vi "Set_reference_Point (SubVI).vi"(7 "Part of multigrid":bool, 8 "error in (no error)":errorcluster, 11 "Application in":refnum<vi>) -> (0 "error out":errorcluster, 3 "Application out":refnum<vi>)   [LabVIEW 2021]
uses:
  <userlib>/Nanonis Prog Interface V5/Nanonis Prog Interface.lvlib
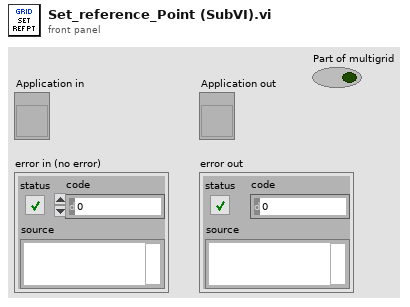
[diagram p1: front panel]
types:
  T1 = cluster{"x(m)":sgl, "y(m)":sgl, "Text":string, "Color":u32}
  T2 = cluster{"X (m)":sgl, "Y (m)":sgl, "Text":string, "Color":u32, "Visible":bool}[]
  T3 = cluster{"X (m)":sgl, "Y (m)":sgl, "Text":string, "Color":u32, "Visible":bool}
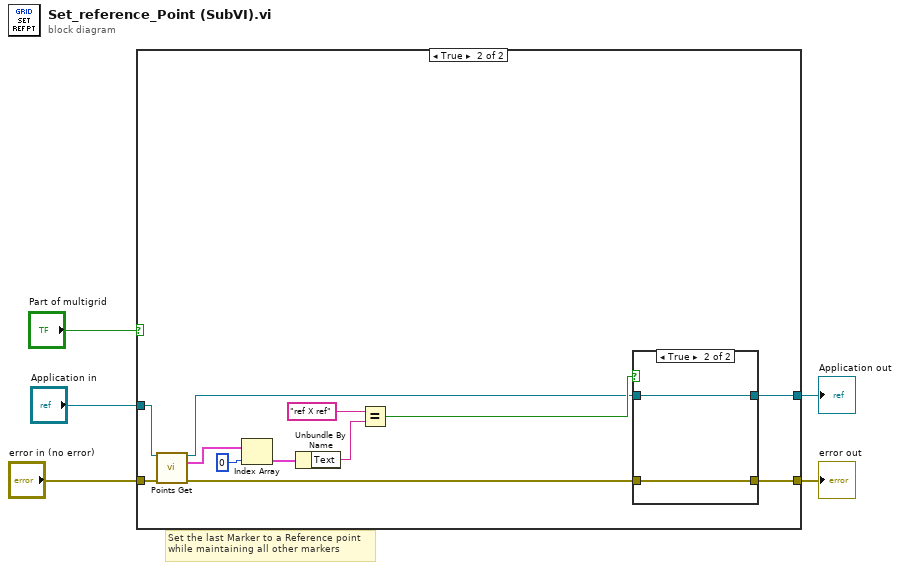
[diagram p0: block diagram]
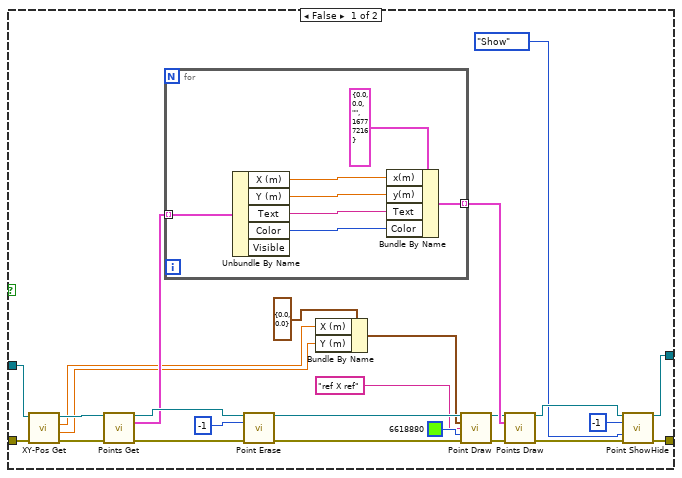
[diagram p2: hidden frame]
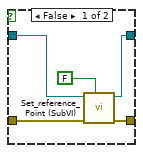
[diagram p3: hidden frame]
diagram:
  # "Set the last Marker to a Reference point\nwhile maintaining all other markers"
  n1 = case shown="True" "Part of multigrid" {
    tunnel: [w20 w38] -> w5
    tunnel: "error in (no error)" -> [w13 w48]
    tunnel: "Application in" -> [w12 w49]
    tunnel: [w6 w39] -> w2
    frame False {
      n2 = call <userlib>:"XY-Pos Get.vi"("error in (no error)"=w13, "Application ref in"=w12) -> ("error out"=w11:errorcluster, "Y (m)"=w19:sgl, "X (m)"=w18:sgl, "Application ref out"=w26:refnum<vi>)  [unwired: 5 in]
      n3 = call <userlib>:"Points Get.vi"("Application ref in"=w26, "error in (no error)"=w11) -> ("Application ref out"=w27:refnum<vi>, "Points"=w25:T2, "error out"=w10:errorcluster)  [unwired: 11 in]
      n4 = for {
        tunnel: w25 -> [w37] mode=indexing
        tunnel: [w31] -> w30 mode=indexing
        n5 = Unbundle By Name(w37) -> ("X (m)"=w35:sgl, "Y (m)"=w34:sgl, "Text"=w33:string, "Color"=w32:u32)  [unwired: 1 out]
        n6 = Bundle By Name(cluster=T1 {"x(m)"=0.0, "y(m)"=0.0, "Text"="", "Color"=16777216} ("Point"), "x(m)"=w35, "y(m)"=w34, "Text"=w33, "Color"=w32) -> (w31:T1)
      }
      n7 = call <userlib>:"Point Erase.vi"("Application ref in"=w27, "Point index (-1=All points)"=-1, "error in (no error)"=w10) -> ("Application ref out"=w23:refnum<vi>, "error out"=w9:errorcluster)  [unwired: 11 in]
      n8 = Bundle By Name(cluster=cluster{"X (m)":sgl, "Y (m)":sgl} {"X (m)"=0.0, "Y (m)"=0.0} ("Point Coordinates"), "X (m)"=w18, "Y (m)"=w19) -> (w17:cluster{"X (m)":sgl, "Y (m)":sgl})
      n9 = call <userlib>:"Point Draw.vi"("Application ref in"=w23, "Point Coordinates"=w17, "Text"="ref X ref", "Color"=u32 6618880, "error in (no error)"=w9) -> ("Application ref out"=w28:refnum<vi>, "error out"=w8:errorcluster)  [unwired: 9 in]
      n10 = call <userlib>:"Points Draw.vi"("Application ref in"=w28, "Points Configuration"=w30, "error in (no error)"=w8) -> ("Application ref out"=w29:refnum<vi>, "error out"=w7:errorcluster)  [unwired: 11 in]
      n11 = call <userlib>:"Point ShowHide.vi"("Application ref in"=w29, "Point index (-1=All points)"=-1, "Show/Hide"=enum16{"Show", "Hide"}."Show", "error in (no error)"=w7) -> ("Application ref out"=w20:refnum<vi>, "error out"=w6:errorcluster)  [unwired: 10 in]
    }
    frame True {
      n12 = call <userlib>:"Points Get.vi"("Application ref in"=w49, "error in (no error)"=w48) -> ("Application ref out"=w41:refnum<vi>, "Points"=w45:T2, "error out"=w40:errorcluster)  [unwired: 11 in]
      n13 = Index Array(array=w45, index=0) -> (element=w43:T3)
      n14 = Unbundle By Name(w43) -> ("Text"=w46:string)
      n15 = Equal?(x="ref X ref" ("Text"), y=w46) -> (x = y?=w42:bool)
      n16 = case shown="True" w42 {
        tunnel: w41 -> [w54 w56]
        tunnel: w40 -> [w53 w55]
        tunnel: [w52 w56] -> w38
        tunnel: [w51 w55] -> w39
        frame False {
          n17 = call "Set_reference_Point (SubVI).vi"("Part of multigrid"=FALSE, "error in (no error)"=w53, "Application in"=w54) -> ("error out"=w51:errorcluster, "Application out"=w52:refnum<vi>)  [unwired: 7 in]
        }
        frame True {
        }
      }
    }
  }
  "error out" <- w2
  "Application out" <- w5
